vi "PH_Beckhoff_PPMA-Rods.ProcCases.vi"(0 "i ref in":refnum<vi>, 1 "selector":string, 2 "Data":T1, 3 "call cluster":T2={"Object"="", "Selector"="", "CallType"=enum."synchronous", "Async Object"="", "Async Selector"="", "Data Descriptor"="", "Data"=[], "Error #"=0, "Expire"=0}, 5 "error in (no error)":errorcluster) -> (14 "i ref out":refnum<vi>, 17 "answer cluster":T2={"Object"="", "Selector"="", "CallType"=enum."synchronous", "Async Object"="", "Async Selector"="", "Data Descriptor"="", "Data"=[], "Error #"=0, "Expire"=0}, 19 "error out":errorcluster)   [LabVIEW 2014, in "PH_Beckhoff_PPMA-Rods.lvlib"]
doc: "This method is called by a process from within the default case in the event loop. The methods of a class that are linked to events will be called from THIS method. Add your code here."
uses:
  PH_Beckhoff_PPMA-Rods.lvlib
  CS_Core/CSSystem/CoreDefs/CoreDefs.call_type.ctl
  CS_Core/BaseProcess/BaseProcess.descriptor string definition.ctl
  CS_Core/CSSystem/CoreDefs/CoreDefs.rawDataType.ctl
  PH_Beckhoff/PH_Beckhoff.lvlib
  CS_Core/BaseProcess/BaseProcess.lvlib
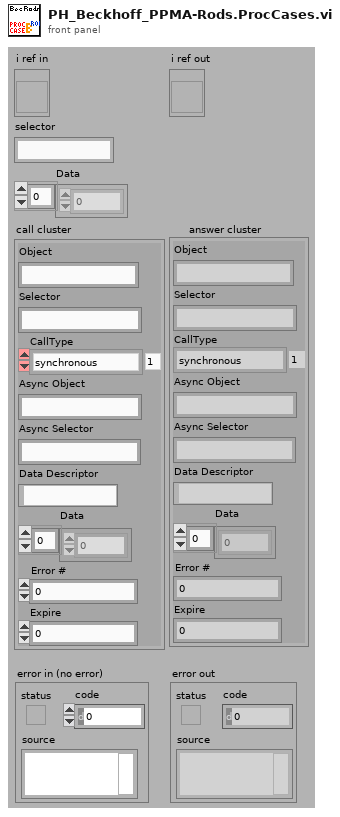
[diagram p1: front panel]
types:
  T1 = typedef "CoreDefs.rawDataType.ctl" = i8[]
  T2 = typedef "CoreDefs.call_type.ctl" = cluster{"Object":string, "Selector":string, "CallType":enum16{"simple", "synchronous", "asynchronous"}, "Async Object":string, "Async Selector":string, "Data Descriptor":T3, "Data":T1, "Error #":i32, "Expire":u32}
  T3 = typedef "BaseProcess.lvlib/BaseProcess.descriptor string definition.ctl" = string
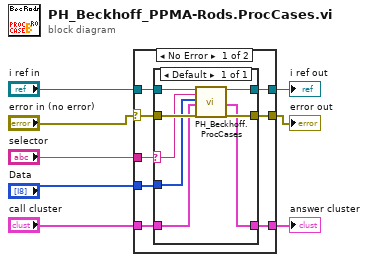
[diagram p0: block diagram]
diagram:
  n1 = case shown="No Error" "error in (no error)" {
    selector: "error in (no error)" -> [w9 w25]
    tunnel: "selector" -> [w16 _]
    tunnel: [w15 w26] -> w7
    tunnel: "Data" -> [w14 _]
    tunnel: "call cluster" -> [w13 w26]
    tunnel: "i ref in" -> [w12 w27]
    tunnel: [w11 w27] -> w3
    tunnel: [w10 w25] -> w2
    frame No Error {
      n2 = case shown="Default" w16 {
        selector: w16 -> [w18]
        tunnel: w14 -> [w19]
        tunnel: w12 -> [w17]
        tunnel: [w24] -> w11
        tunnel: w13 -> [w20]
        tunnel: [w21] -> w15
        tunnel: w9 -> [w23]
        tunnel: [w22] -> w10
        frame Default {
          n3 = call "PH_Beckhoff.ProcCases.vi"("i ref in"=w17, "selector"=w18, "Data"=w19, "call cluster"=w20, "error in (no error)"=w23) -> ("i ref out"=w24:refnum<vi>, "answer cluster"=w21:T2, "error out"=w22:errorcluster)  [unwired: 12 in]
        }
      }
    }
    frame Error {
    }
  }
  "answer cluster" <- w7
  "i ref out" <- w3
  "error out" <- w2
